vi "9601 Error Retrieving Base from Integer String--error.vi"(8 "error in":errorcluster, 11 "Integer String":string) -> (0 "error out":errorcluster)   [LabVIEW 2024, in "Electronic Datasheet.lvlib"]
uses:
  Electronic Datasheet.lvlib
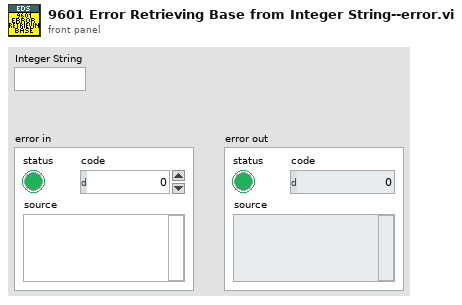
[diagram p1: front panel]
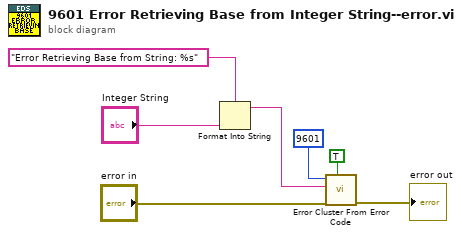
[diagram p0: block diagram]
diagram:
  n1 = Format Into String(format string="Error Retrieving Base from String: %s", "Integer String") -> (resulting string=w4:string)  [unwired: 2 in, 1 out]
  n2 = call <vilib>:"Error Cluster From Error Code.vi"("show call chain? (False)"=TRUE, "error in (no error)"="error in", "error message (\"\")"=w4, "error code (0)"=9601) -> ("error out"=→"error out":errorcluster)  [unwired: 5 in]
